vi "RunTimeMenu Custom Population.vi"(8 "error in (no error)":errorcluster, 10 "Menu Refnum":refnum<k9>, 11 "Node Ptr":u64 format="%.0x") -> (0 "error out":errorcluster)   [LabVIEW 2020, in "Ballard ARINC 429 System Explorer.lvlib"]
uses:
  Ballard ARINC 429 System Explorer.lvlib
  Includes/Ballard ARINC 429 System Explorer.lvlibp/System Explorer/Interfaces/System Explorer Dispatcher/System Explorer Dispatcher.lvclass
  Includes/Ballard ARINC 429 System Explorer.lvlibp/System Explorer/Implementation/System Explorer Dispatcher/System Explorer Dispatcher.lvclass
  C:/git/ni/niveristand-communications-bus-template/Includes/Ballard ARINC 429 System Explorer.lvlibp/System Explorer/Implementation/System Explorer Dispatcher/System Explorer Dispatcher.lvclass
  C:/git/ni/niveristand-communications-bus-template/Includes/Ballard ARINC 429 System Explorer.lvlibp/System Explorer/Interfaces/System Explorer Dispatcher/System Explorer Dispatcher.lvclass
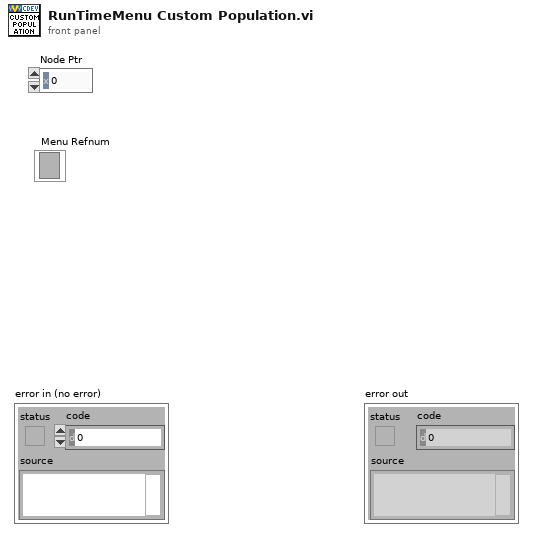
[diagram p1: front panel]
types:
  T1 = typedef "Custom Device API.lvlib/Custom Device Item Ref.ctl" = u64
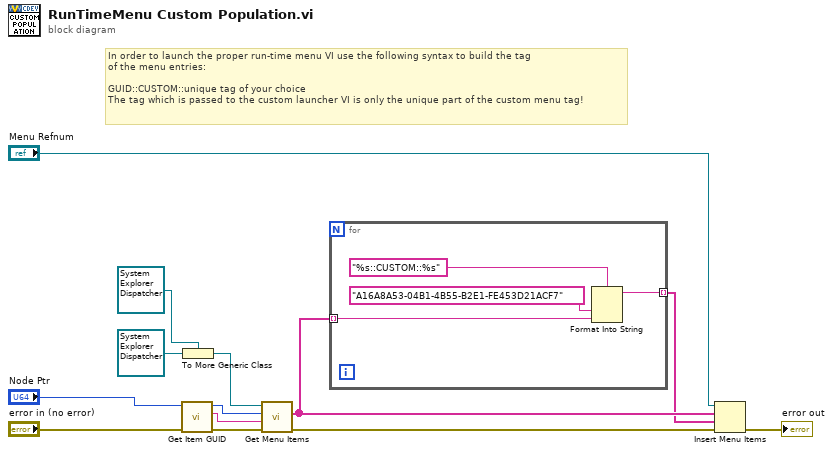
[diagram p0: block diagram]
diagram:
  # "In order to launch the proper run-time menu VI use the following syntax to build the tag\nof the menu entries:\n\nGUID::CUSTOM::unique tag of your choice\nThe tag which is passed to the custom launcher VI is only the unique part of the custom menu tag!"
  n1 = call "Get Item GUID.vi"("error in (no error)"="error in (no error)", "item in"="Node Ptr") -> ("error out"=w6:errorcluster, "guid"=w5:string, "item out"=w8:T1)  [unwired: 7 in]
  n2 = To More Generic Class(target class=refnum<class "System Explorer Dispatcher.lvclass"> refnum ("Ballard ARINC 429 System Explorer.lvlibp:Interfaces.lvlib:System Explorer Dispatcher.lvclass"), reference=refnum<class "System Explorer Dispatcher.lvclass"> refnum ("Ballard ARINC 429 System Explorer.lvlibp:Implementation.lvlib:System Explorer Dispatcher.lvclass")) -> (generic class reference=w11:refnum<class "System Explorer Dispatcher.lvclass">)
  n3 = call-dynamic "Get Menu Items.vi"("error in (no error)"=w6, "GUID"=w5, "Item Ref"=w8, "System Explorer Dispatcher in"=w11) -> ("error out"=w7:errorcluster, "Menu Items"=w4:string[])  [unwired: 5 in, 1 out]
  n4 = for {
    tunnel: w4 -> [w15] mode=indexing
    tunnel: [w14] -> w3 mode=indexing
    n5 = Format Into String(format string="%s::CUSTOM::%s", "A16A8A53-04B1-4B55-B2E1-FE453D21ACF7", w15) -> (resulting string=w14:string)  [unwired: 2 in, 1 out]
  }
  n6 = Insert Menu Items(6:w7, 7:w3, 8:w4, 9:"Menu Refnum") -> (0:→"error out":errorcluster)  [unwired: 2 in, 2 out]
